vi "Read Branch Rate.vi"(8 "error in (no error)":errorcluster, 11 "Coverage in":refnum<class "Coverage.lvclass">) -> (0 "error out":errorcluster, 2 "Branch Rate":dbl, 3 "Coverage out":refnum<class "Coverage.lvclass">)   [LabVIEW 2017, in "Cobertura.lvlib" / "Coverage.lvclass"]
uses:
  Coverage.lvclass
  Coverage.lvclass/Coverage.ctl
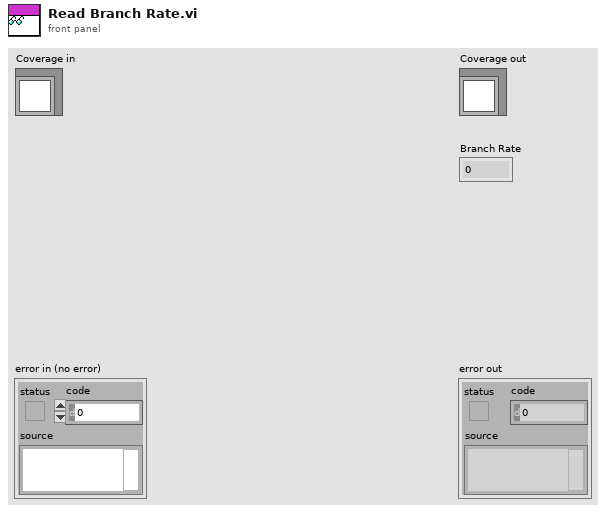
[diagram p1: front panel]
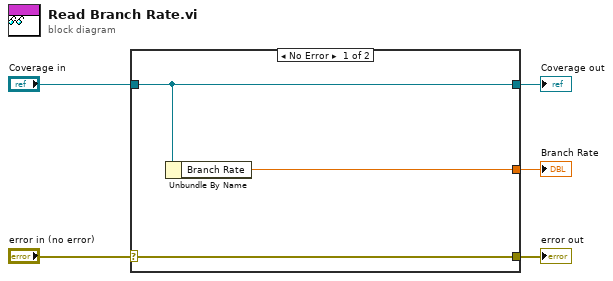
[diagram p0: block diagram]
diagram:
  n1 = case shown="No Error" "error in (no error)" {
    selector: "error in (no error)" -> [w8 w9]
    tunnel: [w8 w9] -> w4
    tunnel: [w7 w10] -> w2
    tunnel: "Coverage in" -> [w7 w10]
    tunnel: [w6 _] -> w1
    frame No Error {
      n2 = Unbundle By Name(w7) -> ("Branch Rate"=w6:dbl)
    }
    frame Error {
    }
  }
  "error out" <- w4
  "Coverage out" <- w2
  "Branch Rate" <- w1
